vi "Write.vi"(8 "error in":errorcluster, 10 "ChillerProducerChannels":T1, 11 "ChillerNew.lvclass":refnum<class "ChillerNew.lvclass">) -> (0 "error out":errorcluster, 3 "output cluster":refnum<class "ChillerNew.lvclass">)   [LabVIEW 2023, in "ChillerNew.lvclass"]
uses:
  ChillerNew.lvclass
  ChillerNew.lvclass/ChillerNew.ctl
  d6de19df-c9e2-43fa-9ac5-572fde5e59f3.vi
  d6de19df-c9e2-43fa-9ac5-572fde5e59f3.vi/4bc1c15b-36ab-481f-b8dd-c64075ce723a.vi
  d6de19df-c9e2-43fa-9ac5-572fde5e59f3.vi/d83cb72b-7713-41fc-a3d1-682de79cf574.vi
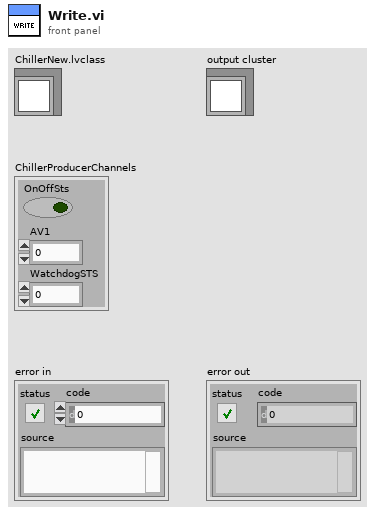
[diagram p1: front panel]
types:
  T1 = cluster{"OnOffSts":bool, "AV1":dbl, "WatchdogSTS":i32}
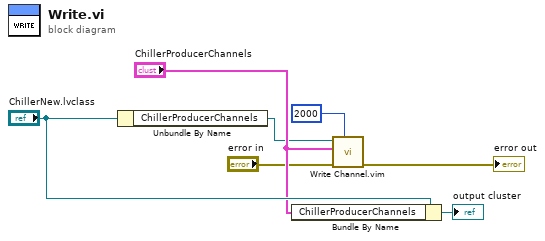
[diagram p0: block diagram]
diagram:
  n1 = Unbundle By Name("ChillerNew.lvclass") -> ("ChillerProducerChannels"=w4:refnum<k21>)
  n2 = Bundle By Name(cluster="ChillerNew.lvclass", "ChillerProducerChannels"="ChillerProducerChannels") -> (→"output cluster":refnum<class "ChillerNew.lvclass">)
  n3 = call "Write Channel.vim"("Timeout (ms)"=2000, "error in"="error in", "Data in"="ChillerProducerChannels", "ADAS HIL Channel in"=w4) -> ("error out"=→"error out":errorcluster)  [unwired: 5 in, 2 out]
